vi "Create Case Structure Frames.vi"(8 "error in (no error)":errorcluster, 10 "Frame Names":string[](array[string]), 11 "CaseStructure in":refnum<vi>) -> (0 "error out":errorcluster, 2 "Case Frames[]":refnum<vi>[](array[refnum]), 3 "CaseStructure out":refnum<vi>)   [LabVIEW 2019, in "VI Scripting Utilities.lvlib"]
uses:
  VI Scripting Utilities.lvlib
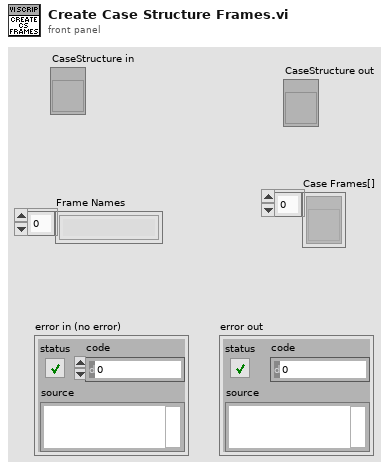
[diagram p1: front panel]
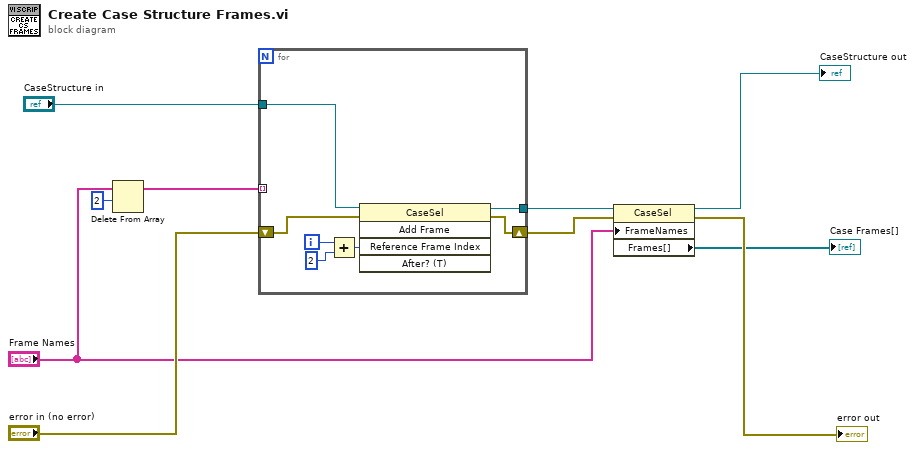
[diagram p0: block diagram]
diagram:
  n1 = Delete From Array(array="Frame Names", length=2) -> (array with subset deleted=w2:string[])  [unwired: 1 in, 1 out]
  n2 = for {
    tunnel: "CaseStructure in" -> [w17]
    tunnel: [w15] -> w8
    shift-right: [w14] -> w5
    shift-left: "error in (no error)" -> [w16]
    tunnel: w2 -> [_] mode=indexing
    i -> [w13]
    n3 = Add(x=w13, y=2) -> (x+y=w11:i32)
    n4 = invoke class="CaseSel" method="Add Frame"(reference=w17, error in=w16, "Reference Frame Index"=w11) -> (reference out=w15:refnum<vi>, error out=w14:errorcluster)  [unwired: 2 in, 3 out]
  }
  n5 = property class="CaseSel"(reference=w8, error in=w5, "FrameNames"="Frame Names") -> (reference out=→"CaseStructure out":refnum<vi>, error out=→"error out":errorcluster, "Frames[]"=→"Case Frames[]":refnum<vi>[])
